vi "Add Error.vi"(8 "error in (no error)":errorcluster, 9 "String to Append":string, 11 "Insert Error":bool=TRUE) -> (0 "error out":errorcluster)   [LabVIEW 2021, in "CIF_NIChn_Fifo_Power_DVR.lvclass"]
uses:
  CIF_NIChn_Fifo_Power_DVR.lvclass
  CIF_NIChn_Fifo_Power_DVR.lvclass/CIF_NIChn_Fifo_Power_DVR.ctl
  CIFCore/Common/CIFCoreCommon.lvlib
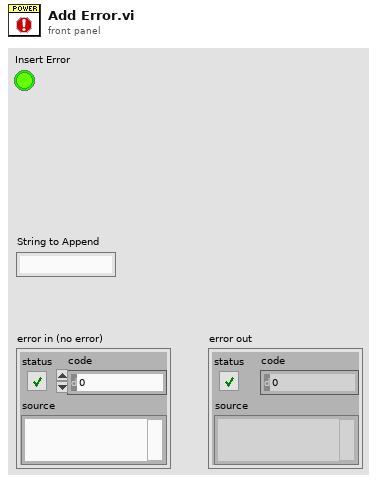
[diagram p1: front panel]
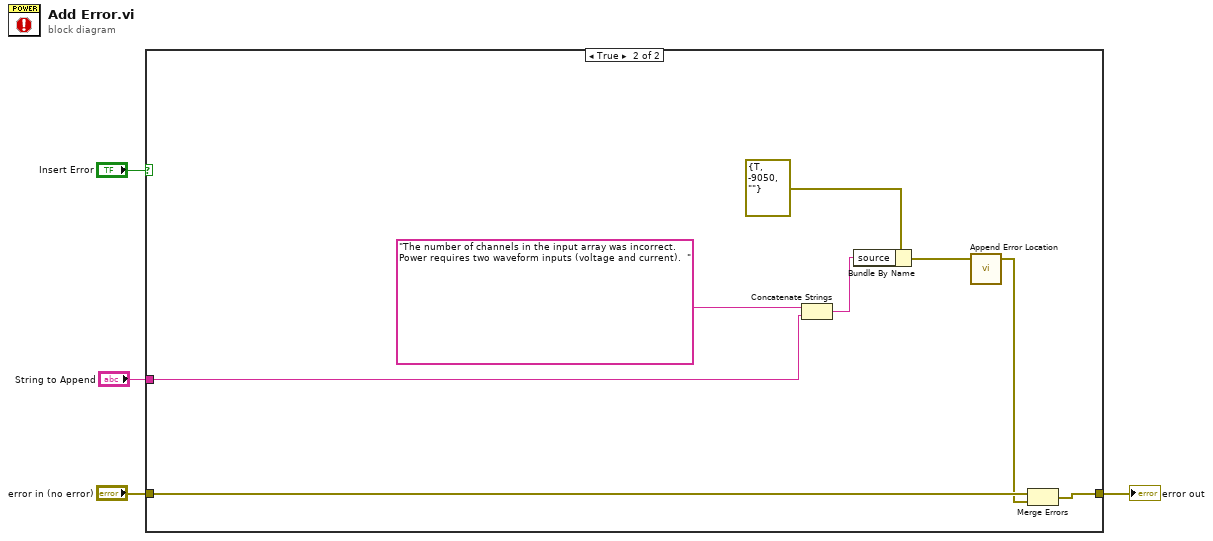
[diagram p0: block diagram]
diagram:
  n1 = case shown="True" "Insert Error" {
    tunnel: [w5 w11] -> w3
    tunnel: "error in (no error)" -> [w5 w12]
    tunnel: "String to Append" -> [_ w13]
    frame False {
    }
    frame True {
      n2 = Concatenate Strings("The number of channels in the input array was incorrect.  Power requires two waveform inputs (voltage and current).  " ("source"), w13) -> (w7:string)
      n3 = Bundle By Name(cluster=errorcluster {"status"=TRUE, "code"=-9050, "source"=""} ("Invalid ID"), "source"=w7) -> (w10:errorcluster)
      n4 = call "Append Error Location.vi"("error in (no error)"=w10) -> ("error out"=w9:errorcluster)  [unwired: 4 in]
      n5 = Merge Errors(w12, w9) -> (w11:errorcluster)
    }
  }
  "error out" <- w3
